vi "Start Log.vi"(8 "error in (no error)":errorcluster, 9 "Timestamp":string, 10 "Series":string, 11 "LoggingManager in":refnum<class "LoggingManager.lvclass">) -> (0 "error out":errorcluster, 3 "LoggingManager out":refnum<class "LoggingManager.lvclass">)   [LabVIEW 2020, in "VolatusDataLogger.lvlib" / "LoggingManager.lvclass"]
uses:
  LoggingManager.lvclass
  C:/dev/lv20CE/relink/lv-volatus/Volatus/Task/Task.lvclass
  LoggingManager.lvclass/LoggingManager.ctl
  Volatus/Task/Task.lvclass/Task.ctl
  Volatus/Event API/EventAPI.lvclass/EventAPI.ctl
  Volatus/EventHandler Messages/Handle Event Msg/Handle Event Msg.lvclass/Handle Event Msg.ctl
  <vilib>/ActorFramework/Message Enqueuer/Message Enqueuer.lvclass/Message Enqueuer.ctl
  LoggingManager Messages/Start Log Msg/Start Log Msg.lvclass/Start Log Msg.ctl
  <vilib>/ActorFramework/Message Enqueuer/Enqueue.vi
  Volatus/EventHandler Messages/Handle Event Msg/Send Handle Event.vi
  Volatus/EventHandler Messages/Handle Event Msg/Handle Event Msg.lvclass
  C:/Program Files (x86)/National Instruments/LabVIEW 2020/vi.lib/ActorFramework/Message/Message.lvclass
  LoggingManager Messages/Start Log Msg/Start Log Msg.lvclass
  Volatus/Task/Task ID.vi
  <vilib>/ActorFramework/Message Priority Queue/Priority Enqueue.vi
  Volatus/Task/Task.lvclass
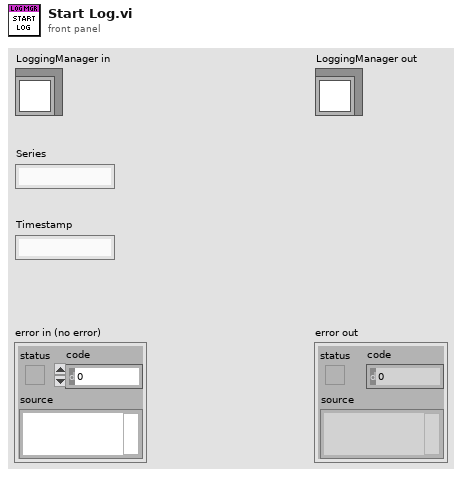
[diagram p1: front panel]
types:
  T1 = map{string, refnum<class "Message Enqueuer.lvclass">}
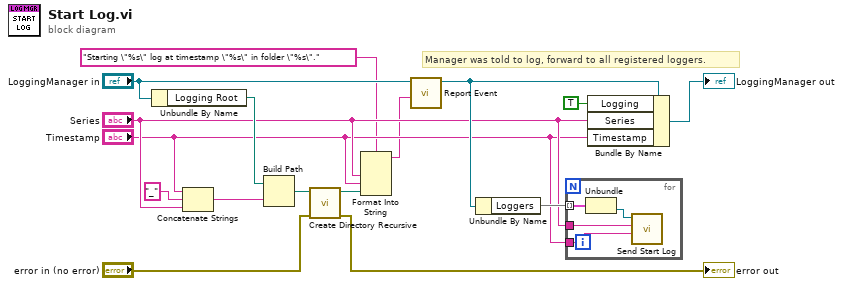
[diagram p0: block diagram]
diagram:
  # "Manager was told to log, forward to all registered loggers."
  n1 = Unbundle By Name("LoggingManager in") -> ("Logging Root"=w10:path)
  n2 = Concatenate Strings("Timestamp", "_" ("string"), "Series") -> (w12:string)
  n3 = Build Path(base path=w10, name or relative path=w12) -> (appended path=w9:path)
  n4 = call <vilib>:"Create Directory Recursive.vi"("error in (no error)"="error in (no error)", "directory"=w9) -> ("error out"=→"error out":errorcluster, "directory copy"=w5:path)  [unwired: 3 in, 1 out]
  n5 = Format Into String(format string="Starting \"%s\" log at timestamp \"%s\" in folder \"%s\".", "Series", "Timestamp", w5) -> (resulting string=w1:string)  [unwired: 2 in, 1 out]
  n6 = call "Report Event.vi"("Message"=w1, "Task in"="LoggingManager in") -> ("Task out"=w6:refnum<class "LoggingManager.lvclass">)  [unwired: 8 in, 1 out]
  n7 = Unbundle By Name(w6) -> ("Loggers"=w16:T1)
  n8 = for {
    tunnel: w16 -> [w20] mode=indexing
    tunnel: "Series" -> [w19]
    tunnel: "Timestamp" -> [w18]
    n9 = Unbundle(w20) -> ("EnQr"=w17:refnum<class "Message Enqueuer.lvclass">)  [unwired: 1 out]
    n10 = call "Send Start Log.vi"("Timestamp"=w18, "Series"=w19, "Message Enqueuer"=w17) -> ()  [unwired: 7 in, 2 out]
  }
  n11 = Bundle By Name(cluster=w6, "Logging"=TRUE, "Series"="Series", "Timestamp"="Timestamp") -> (→"LoggingManager out":refnum<class "LoggingManager.lvclass">)
